vi "Insert Element at Index.vi"(6 "index":i32, 8 "error in (no error)":errorcluster, 9 "element":variant, 10 "Name":string, 11 "Variant in":variant) -> (0 "error out":errorcluster, 3 "Variant out":variant)   [LabVIEW 2017, in "Advanced Variant Tools.lvlib" / "Cluster Manipulation.lvlib"]
uses:
  Cluster Manipulation.lvlib
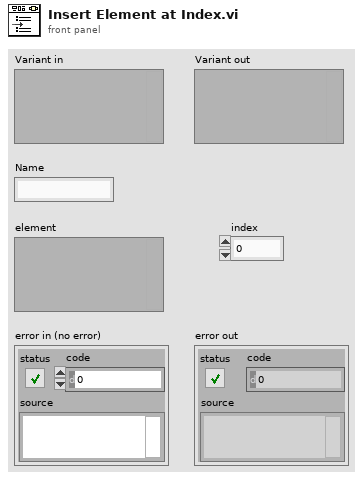
[diagram p1: front panel]
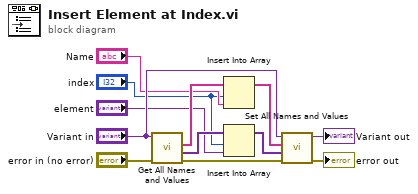
[diagram p0: block diagram]
diagram:
  n1 = call "Get All Names and Values.vi"("error in"="error in (no error)", "Cluster In"="Variant in") -> ("error out"=w11:errorcluster, "Values"=w4:variant[], "Names"=w7:string[])  [unwired: 6 in, 1 out]
  n2 = Insert Into Array(array=w7, index="index", new element="Name") -> (w5:string[])
  n3 = Insert Into Array(array=w4, index="index", new element="element") -> (w1:variant[])
  n4 = call "Set All Names and Values.vi"("error in"=w11, "values"=w1, "Names"=w5, "Cluster In"="Variant in") -> ("error out"=→"error out":errorcluster, "Cluster Out"=→"Variant out":variant)  [unwired: 6 in]
